vi "Walsh Hadamard Inverse PtByPt.vi"(2 "initialize":bool, 3 "sample length":i32=100, 5 "x":dbl format="%0.2f") -> (0 "error":i32, 1 "Walsh Hadamard Inverse {X}":dbl[](array[numeric]))   [LabVIEW 2017, in "NI_PtbyPt.lvlib"]
doc: "Performs the inverse of the real Walsh Hadamard transform."
uses:
  <vilib>/ptbypt/NI_PtbyPt.lvlib
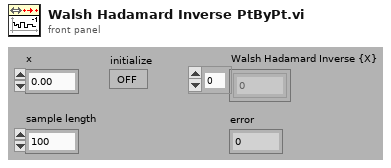
[diagram p1: front panel]
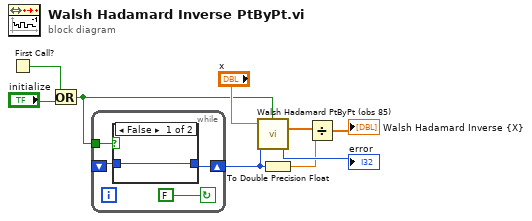
[diagram p0: block diagram]
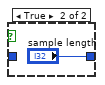
[diagram p2: hidden frame]
diagram:
  n1 = First Call?() -> (First Call?: T/F=w3:bool)
  n2 = Or(x=w3, y="initialize") -> (x .or. y?=w2:bool)
  n3 = while {
    shift-left: _ -> [w11]
    shift-right: [w12] -> w1
    tunnel: w2 -> [w13]
    stop <- FALSE continue-if-true
    n4 = case shown="False" w13 {
      tunnel: [w14 "sample length"] -> w12
      tunnel: w11 -> [w14 _]
      frame False {
      }
      frame True {
      }
    }
  }
  n5 = call <vilib>:"Walsh Hadamard PtByPt (obs 85).vi"("initialize"=w2, "sample length"=w1, "x"="x") -> ("error"=→"error":i32, "Walsh Hadamard {X}"=w9:dbl[])  [unwired: 1 in]
  n6 = To Double Precision Float(number=w1) -> (double precision float=w5:dbl)
  n7 = Divide(x=w9, y=w5) -> (x/y=→"Walsh Hadamard Inverse {X}":dbl[])
